vi "GEOM_findReadMode.vi"(9 "binning corrected?":bool=TRUE, 10 "GEOM_FPAReadModes":T3[](array[typedef]) {"Amplifiers"."fliped" items=["none", "horizontal", "vertical"]; "Amplifiers"."type" items=["LL", "LR", "UL", "UR"]}, 11 "readmode":string) -> (0 "corramp found":bool, 1 "BinFPA":T2, 2 "FPAReadMode":T3 {"Amplifiers"."fliped" items=["none", "horizontal", "vertical"]; "Amplifiers"."type" items=["LL", "LR", "UL", "UR"]}, 3 "amp found":bool, 4 "detreadmode":cluster{"name":string, "detectors":T1[]}, 6 "det found":bool)   [LabVIEW 2016]
uses:
  GEOM_FPAReadMode.ctl
  GEOM_Amplifier.ctl
  GEOM_AmpType.ctl
  GEOM_ROI.ctl
  GEOM_Coords.ctl
  GEOM_CorrectedFPA.ctl
  GEOM_DetSummaryStruct.ctl
  GEOM_VAR_action.ctl
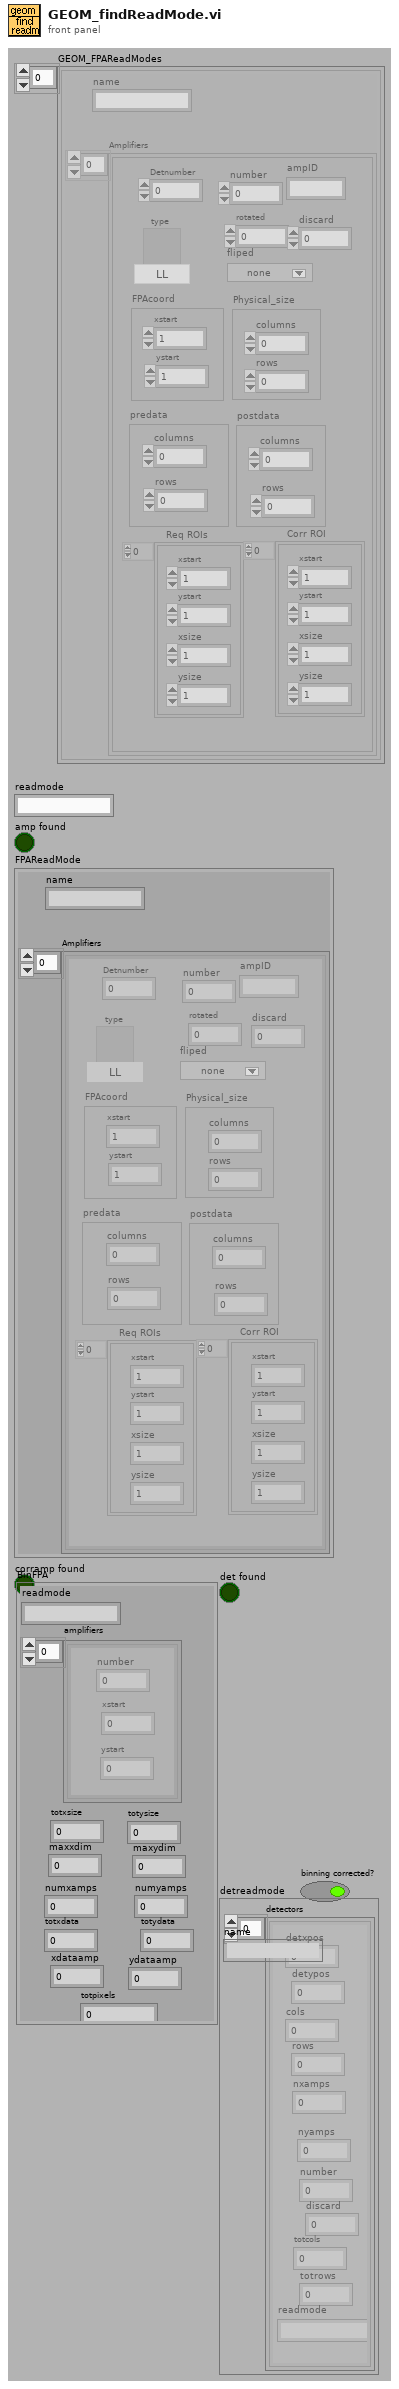
[diagram p1: front panel]
types:
  T1 = typedef "GEOM_DetSummaryStruct.ctl" = cluster{"detxpos":i32, "detypos":i32, "cols":i32, "rows":i32, "nxamps":i32, "nyamps":i32, "number":i32, "discard":i32, "totcols":i32, "totrows":i32, "readmode":string}
  T2 = typedef "GEOM_CorrectedFPA.ctl" = cluster{"readmode":string, "amplifiers":cluster{"number":i32, "xstart":i32, "ystart":i32}[], "totxsize":i32, "totysize":i32, "maxxdim":i32, "maxydim":i32, "numxamps":i32, "numyamps":i32, "totxdata":i32, "totydata":i32, "xdataamp":i32, "ydataamp":i32, "totpixels":i32}
  T3 = typedef "GEOM_FPAReadMode.ctl" = cluster{"name":string, "Amplifiers":T4[]}
  T4 = typedef "GEOM_Amplifier.ctl" = cluster{"number":i32, "type":T5, "rotated":i16, "fliped":u16, "FPAcoord":cluster{"xstart":i32, "ystart":i32}, "Physical_size":cluster{"columns":i32, "rows":i32}, "predata":cluster{"columns":i32, "rows":i32}, "postdata":cluster{"columns":i32, "rows":i32}, "Req ROIs":T6, "Corr ROI":T6, "Detnumber":i32, "ampID":string, "discard":i32}
  T5 = typedef "GEOM_AmpType.ctl" = u16
  T6 = typedef "GEOM_ROI.ctl" = T7[]
  T7 = typedef "GEOM_Coords.ctl" = cluster{"xstart":u32, "ystart":u32, "xsize":u32, "ysize":u32}
  T8 = typedef "GEOM_VAR_action.ctl" = enum16{"read", "write"}
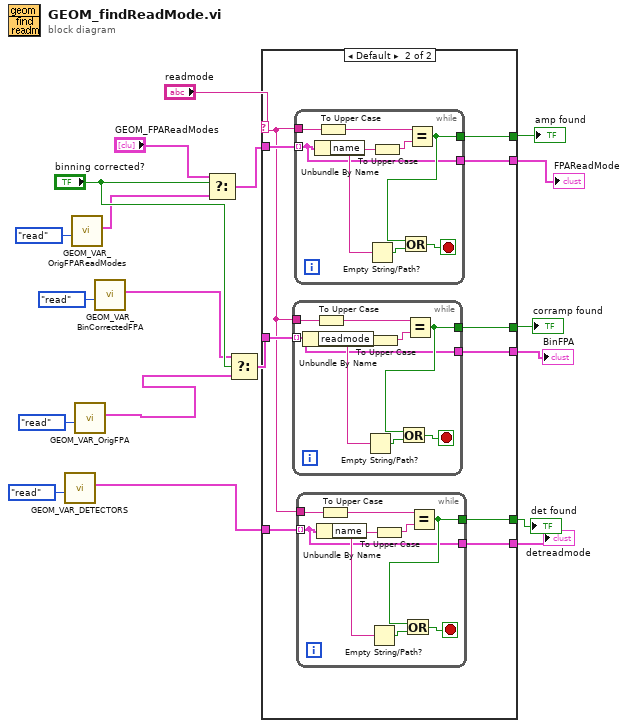
[diagram p0: block diagram]
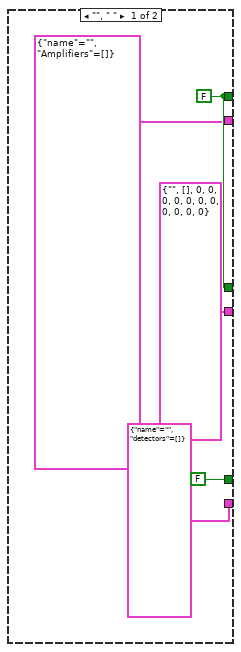
[diagram p2: hidden frame]
diagram:
  n1 = call "GEOM_VAR_DETECTORS.vi"("Action"=GEOM_VAR_action."read") -> ("det out"=w3:cluster{"name":string, "detectors":T1[]}[])  [unwired: 1 in, 9 out]
  n2 = call "GEOM_VAR_OrigFPAReadModes.vi"("Action"=GEOM_VAR_action."read") -> ("GEOM_OrigFPAReadModes out"=w6:T3[])  [unwired: 1 in, 9 out]
  n3 = call "GEOM_VAR_OrigFPA.vi"("Action"=GEOM_VAR_action."read") -> ("GEOM_OrigFPA  out"=w8:T2[])  [unwired: 1 in, 9 out]
  n4 = call "GEOM_VAR_BinCorrectedFPA.vi"("Action"=GEOM_VAR_action."read") -> ("GEOM_BinCorrectedFPA out"=w10:T2[])  [unwired: 1 in, 9 out]
  n5 = Select(t="GEOM_FPAReadModes", s="binning corrected?", f=w6) -> (s? t:f=w13:T3[])
  n6 = Select(t=w10, s="binning corrected?", f=w8) -> (s? t:f=w12:T2[])
  n7 = case shown="Default" "readmode" {
    selector: "readmode" -> [_ w27]
    tunnel: w13 -> [_ w34]
    tunnel: [w24 w33] -> w19
    tunnel: [T3 {"name"="", "Amplifiers"=[]} ("FPAReadMode") w32] -> w18
    tunnel: w12 -> [_ w31]
    tunnel: [w24 w30] -> w17
    tunnel: [T2 {"readmode"="", "amplifiers"=[], "totxsize"=0, "totysize"=0, "maxxdim"=0, "maxydim"=0, "numxamps"=0, "numyamps"=0, "totxdata"=0, "totydata"=0, "xdataamp"=0, "ydataamp"=0, "totpixels"=0} ("GEOM_BinCorrectedFPA") w29] -> w16
    tunnel: w3 -> [_ w28]
    tunnel: [FALSE w26] -> w2
    tunnel: [cluster{"name":string, "detectors":T1[]} {"name"="", "detectors"=[]} ("detreadmodes") w25] -> w1
    frame "", " " {
      w24 = FALSE
    }
    frame Default {
      n8 = while {
        tunnel: w31 -> [w44] mode=indexing
        tunnel: w27 -> [w50]
        tunnel: [w45] -> w30
        tunnel: [w44] -> w29
        stop <- w47 stop-if-true
        n9 = Unbundle By Name(w44) -> ("readmode"=w46:string)
        n10 = To Upper Case(1:w50) -> (0:w49:string)
        n11 = Empty String/Path?(string/path=w46) -> (empty?=w43:bool)
        n12 = To Upper Case(1:w46) -> (0:w48:string)
        n13 = Equal?(x=w49, y=w48) -> (x = y?=w45:bool)
        n14 = Or(x=w45, y=w43) -> (x .or. y?=w47:bool)
      }
      n15 = while {
        tunnel: w34 -> [w52] mode=indexing
        tunnel: w27 -> [w58]
        tunnel: [w53] -> w33
        tunnel: [w52] -> w32
        stop <- w55 stop-if-true
        n16 = Unbundle By Name(w52) -> ("name"=w54:string)
        n17 = To Upper Case(1:w58) -> (0:w57:string)
        n18 = Empty String/Path?(string/path=w54) -> (empty?=w51:bool)
        n19 = To Upper Case(1:w54) -> (0:w56:string)
        n20 = Equal?(x=w57, y=w56) -> (x = y?=w53:bool)
        n21 = Or(x=w53, y=w51) -> (x .or. y?=w55:bool)
      }
      n22 = while {
        tunnel: w28 -> [w36] mode=indexing
        tunnel: w27 -> [w42]
        tunnel: [w37] -> w26
        tunnel: [w36] -> w25
        stop <- w39 stop-if-true
        n23 = Unbundle By Name(w36) -> ("name"=w38:string)
        n24 = To Upper Case(1:w42) -> (0:w41:string)
        n25 = Empty String/Path?(string/path=w38) -> (empty?=w35:bool)
        n26 = To Upper Case(1:w38) -> (0:w40:string)
        n27 = Equal?(x=w41, y=w40) -> (x = y?=w37:bool)
        n28 = Or(x=w37, y=w35) -> (x .or. y?=w39:bool)
      }
    }
  }
  "amp found" <- w19
  "FPAReadMode" <- w18
  "corramp found" <- w17
  "BinFPA" <- w16
  "det found" <- w2
  "detreadmode" <- w1
